vi "HandleItemActivation.vi"(8 "error in (no error)":errorcluster, 11 "ProjectWizardClickableText in":refnum<class "ProjectWizardClickableText.lvclass">) -> (0 "error out":errorcluster, 3 "ProjectWizardClickableText out":refnum<class "ProjectWizardClickableText.lvclass">)   [LabVIEW 2009, in "NavScreen.lvlib" / "ProjectWizardClickableText.lvclass"]
uses:
  ProjectWizardClickableText.lvclass
  ProjectWizardClickableText.lvclass/ProjectWizardClickableText.ctl
  ProjectWizard/ProjectWizard.lvclass
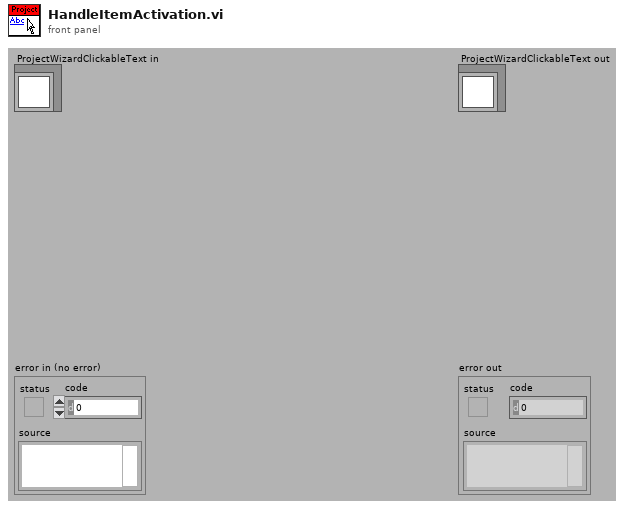
[diagram p1: front panel]
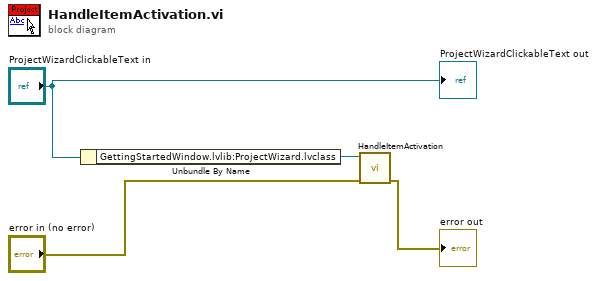
[diagram p0: block diagram]
diagram:
  n1 = Unbundle By Name("ProjectWizardClickableText in") -> ("GettingStartedWindow.lvlib:ProjectWizard.lvclass"=w4:refnum<class "ProjectWizard.lvclass">)
  n2 = call "HandleItemActivation.vi"("error in (no error)"="error in (no error)", "GettingStartedWindow.lvlib:ProjectWizard.lvclass"=w4) -> ("error out"=→"error out":errorcluster)  [unwired: 8 in, 1 out]
  "ProjectWizardClickableText out" <- "ProjectWizardClickableText in"
